vi "Ke2000 Reading.vi"(8 "error in (no error)":errorcluster, 11 "VISA resource name":refnum<visa-resource-name>) -> (0 "error out":errorcluster, 1 "Units":string, 2 "Measurement":dbl, 3 "VISA resource name out":refnum<visa-resource-name>)   [LabVIEW 2009]
panel:
  out "Channel":i32
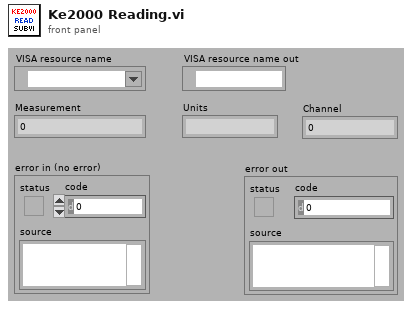
[diagram p1: front panel]
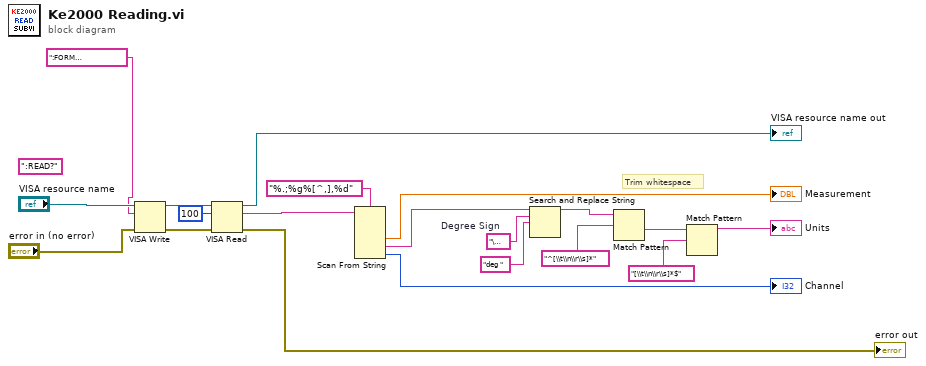
[diagram p0: block diagram]
diagram:
  (unwired) ":READ?" ("write buffer")
  w6 = "\u0013"  # Degree Sign
  # "Trim whitespace"
  n1 = VISA Write(VISA resource name="VISA resource name", write buffer=":FORM ASC;:FORM:ELEM READ,UNIT,CHAN;:SENS:DATA?", error in (no error)="error in (no error)") -> (VISA resource name out=w20:refnum<visa-resource-name>, error out=w19:errorcluster)  [unwired: 1 out]
  n2 = VISA Read(VISA resource name=w20, byte count=u32 100, error in (no error)=w19) -> (VISA resource name out=→"VISA resource name out":refnum<visa-resource-name>, read buffer=w4:string, error out=→"error out":errorcluster)  [unwired: 1 out]
  n3 = Scan From String(format string="%.;%g%[^,],%d", input string=w4) -> (output 1=→"Measurement":dbl, output 2=w7:string, output 3=→"Channel":i32)  [unwired: 5 in, 3 out]
  n4 = Search and Replace String(input string=w7, search string=w6, replace string="deg " ("replace string (\"\")")) -> (result string=w14:string)  [unwired: 5 in, 3 out]
  n5 = Match Pattern(string=w14, regular expression="^[\\t\\n\\r\\s]*") -> (after substring=w11:string)  [unwired: 1 in, 3 out]
  n6 = Match Pattern(string=w11, regular expression="[\\t\\n\\r\\s]*$") -> (before substring=→"Units":string)  [unwired: 1 in, 3 out]
